vi "Rolling Average Array.vi"(0 "Raw Signals":dbl[](array[numeric]), 7 "Rolling Average Size":i32=10 min=1 step=1, 11 "Trim HI / LO [%]":dbl=2.0 min=0.0 max=100.0) -> (4 "Averaged Signals":dbl[](array[numeric]))   [LabVIEW 2012]
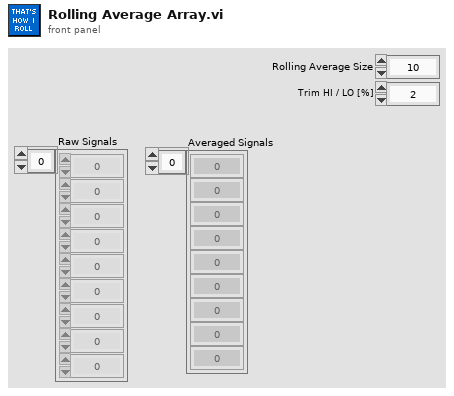
[diagram p1: front panel]
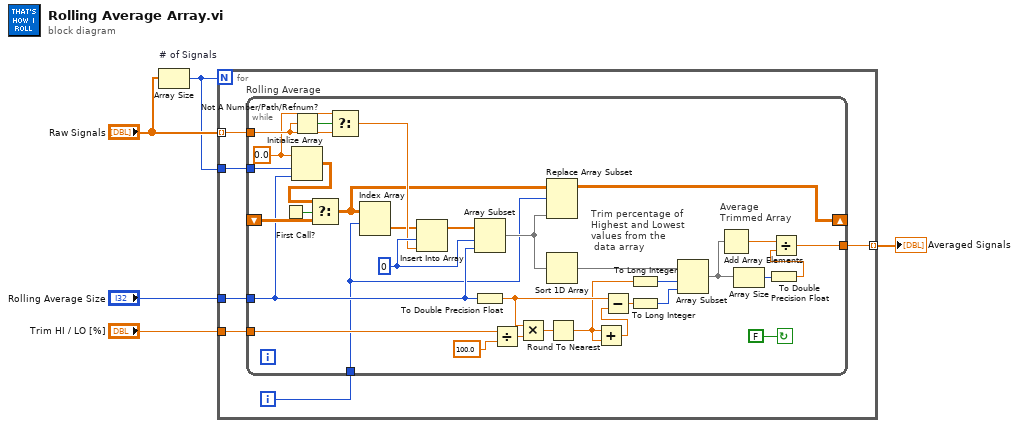
[diagram p0: block diagram]
diagram:
  n1 = Array Size "# of Signals"(array="Raw Signals") -> (size(s)=w2:i32)
  n2 = for {
    N: w2 -> [_]
    tunnel: [w11] -> w5 mode=indexing
    tunnel: "Raw Signals" -> [w9] mode=indexing
    tunnel: w2 -> [w8]
    tunnel: "Rolling Average Size" -> [w7]
    tunnel: "Trim HI / LO [%]" -> [w6]
    i -> [w10]
    n3 = while "Rolling Average" {
      tunnel: w9 -> [w43]
      tunnel: w7 -> [w14]
      shift-right: [w36] -> _
      shift-left: _ -> [w34]
      tunnel: [w15] -> w11
      tunnel: w10 -> [w12]
      tunnel: w8 -> [w31]
      tunnel: w6 -> [w13]
      stop <- FALSE continue-if-true
      w38 = 0.0
      w41 = 0
      # "Average\nTrimmed Array"
      # "Trim percentage of\nHighest and Lowest\nvalues from the\n data array"
      n4 = First Call?() -> (First Call?: T/F=w40:bool)
      n5 = Not A Number/Path/Refnum?(number/path/refnum=w43) -> (NaN/Path/Refnum?=w39:bool)
      n6 = Initialize Array(w38, w31, w14) -> (w32:dbl[][])
      n7 = Select(t=w32, s=w40, f=w34) -> (s? t:f=w33:dbl[][])
      n8 = Select(t=w38, s=w39, f=w43) -> (s? t:f=w37:dbl)
      n9 = Index Array(array=w33, index (row)=w12) -> (element=w35:dbl[])  [unwired: 1 in]
      n10 = Insert Into Array(array=w35, index=w41, new element=w37) -> (w42:dbl[])
      n11 = Array Subset(array=w42, index=w41, length=w14) -> (w17:dbl[])
      n12 = To Double Precision Float(number=w14) -> (double precision float=w25:dbl)
      n13 = Divide(x=w13, y=100.0) -> (x/y=w26:dbl)
      n14 = Multiply(x=w25, y=w26) -> (x*y=w19:dbl)
      n15 = Replace Array Subset(array=w33, new element=w17, index (row)=w12) -> (w36:dbl[][])  [unwired: 1 in]
      n16 = Sort 1D Array(array=w17) -> (sorted array=w23:dbl[])
      n17 = Round To Nearest(number=w19) -> (nearest integer value=w20:dbl)
      n18 = Add(x=w20, y=w20) -> (x+y=w24:dbl)
      n19 = Subtract(x=w25, y=w24) -> (x-y=w18:dbl)
      n20 = To Long Integer(number=w20) -> (32bit integer=w22:i32)
      n21 = To Long Integer(number=w18) -> (32bit integer=w21:i32)
      n22 = Array Subset(array=w23, index=w22, length=w21) -> (w30:dbl[])
      n23 = Add Array Elements(numeric array=w30) -> (sum=w28:dbl)
      n24 = Array Size(array=w30) -> (size(s)=w27:i32)
      n25 = To Double Precision Float(number=w27) -> (double precision float=w16:dbl)
      n26 = Divide(x=w28, y=w16) -> (x/y=w15:dbl)
    }
  }
  "Averaged Signals" <- w5
